vi "Swerve Drive Configs.vi"(0 "Ramp Rate":sgl, 1 "PID Constants":T1={"P Gain"=0.0, "I Gain"=0.0, "D Gain"=0.0, "F Gain"=0.0, "I Zone"=0.0, "Min Output"=-1.0, "Max Output"=1.0}, 2 "Input IDs":T4, 3 "Inversions?":T3, 4 "Idle Mode":T2) -> ()   [LabVIEW 2020]
doc: "A quick bundle to initialize all Swerve Steer motors. \nFUTURE NOTE: Consider adding individual PID controls based on performance."
uses:
  <vilib>/Rock Robotics/WPI/ThirdParty/REV Robotics/REVLib/Typedef/Spark MAX Idle Mode.ctl
  <vilib>/Rock Robotics/WPI/ThirdParty/REV Robotics/REVLib/Typedef/Spark MAX Motor Type.ctl
  <vilib>/Rock Robotics/WPI/ThirdParty/REV Robotics/REVLib/Typedef/Spark MAX Sensor Type.ctl
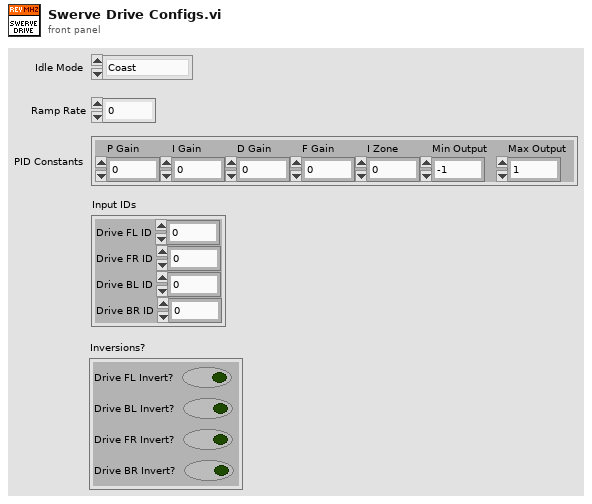
[diagram p1: front panel]
types:
  T1 = cluster{"P Gain":dbl, "I Gain":dbl, "D Gain":dbl, "F Gain":dbl, "I Zone":dbl, "Min Output":dbl, "Max Output":dbl}
  T2 = typedef "Spark MAX Idle Mode.ctl" = enum16{"Coast", "Brake"}
  T3 = cluster{"Drive FL Invert?":bool, "Drive BL Invert?":bool, "Drive FR Invert?":bool, "Drive BR Invert?":bool}
  T4 = cluster{"Drive FL ID":u8, "Drive FR ID":u8, "Drive BL ID":u8, "Drive BR ID":u8}
  T5 = typedef "Spark MAX Sensor Type.ctl" = enum16{"No Sensor", "Hall Sensor", "Encoder", "-Not Available-", "Analog", "Alternate Encoder", "Duty Cycle"}
  T6 = typedef "Spark MAX Motor Type.ctl" = enum16{"Brushed", "Brushless"}
  T7 = typedef "WPI_MotorControlDeviceRef.ctl" = cluster{"DeviceStatus":errorcluster, "Type":T8, "PWM":cluster{"PWM Channel":T9, "DeadBand":T10}, "CAN":cluster{"Device Number":u8, "SetOutput VI Ref":variant, "GetOutput VI Ref":variant, "Enable VI Ref":variant, "Disable VI Ref":variant, "Data":variant}, "Invert":bool, "DIO PWM":cluster{"PWM \"Enable\" Channel":T9, "DIOChannel":T11, "PWM Rate":dbl}}
  T8 = typedef "WPI_MotorControlType.ctl" = enum16{"PWM", "CAN", "DIO PWM"}
  T9 = typedef "FPGA_DIOPWMChannel.ctl" = enum8{"PWM 0", "PWM 1", "PWM 2", "PWM 3", "PWM 4", "PWM 5", "PWM 6", "PWM 7", "PWM 8", "PWM 9", "PWM MXP 0", "PWM MXP 1", "PWM MXP 2", "PWM MXP 3", "PWM MXP 4", "PWM MXP 5", "PWM MXP 6", "PWM MXP 7", "PWM MXP 8", "PWM MXP 9", "Invalid"}
  T10 = typedef "WPI_PWMDeadband.ctl" = cluster{"Name":string, "maxPositivePwm":i32, "minPositivePwm":i32, "centerPwm":i32, "maxNegativePwm":i32, "minNegativePwm":i32, "angularRange":u16}
  T11 = typedef "FPGA_DIOChannel.ctl" = enum8{"DIO 0", "DIO 1", "DIO 2", "DIO 3", "DIO 4", "DIO 5", "DIO 6", "DIO 7", "DIO 8", "DIO 9", "DIO MXP 0", "DIO MXP 1", "DIO MXP 2", "DIO MXP 3", "DIO MXP 4", "DIO MXP 5", "DIO MXP 6", "DIO MXP 7", "DIO MXP 8", "DIO MXP 9", "DIO MXP 10", "DIO MXP 11", "DIO MXP 12", "DIO MXP 13", "DIO MXP 14", "DIO MXP 15", "SPI Port CS1", "SPI Port CS2", "SPI Port CS3", "SPI Port MISO", "SPI Port MOSI", "Invalid"}
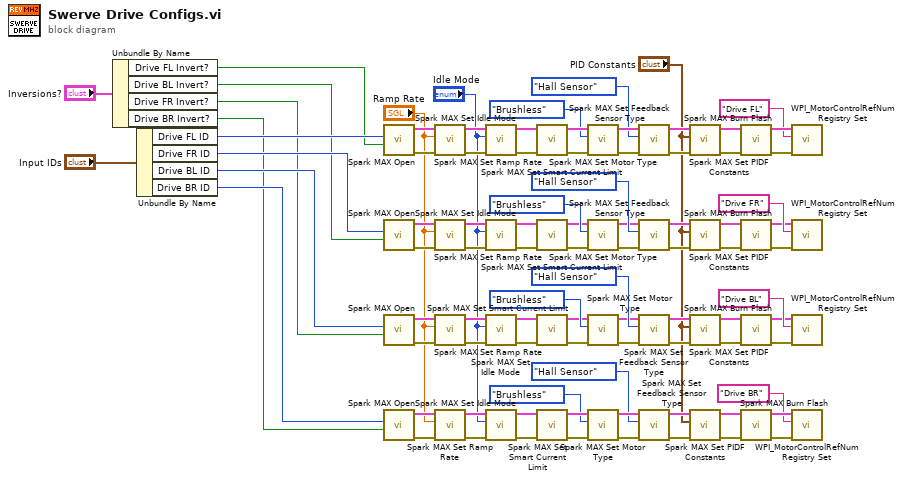
[diagram p0: block diagram]
diagram:
  n1 = Unbundle By Name("Inversions?") -> ("Drive FL Invert?"=w78:bool, "Drive BL Invert?"=w6:bool, "Drive FR Invert?"=w5:bool, "Drive BR Invert?"=w4:bool)
  n2 = Unbundle By Name("Input IDs") -> ("Drive FL ID"=w80:u8, "Drive FR ID"=w9:u8, "Drive BL ID"=w8:u8, "Drive BR ID"=w7:u8)
  n3 = call <vilib>:"Spark MAX Open.vi"("Invert"=w78, "Device Number"=w80) -> ("error out"=w67:errorcluster, "MotorControlDeviceRef"=w68:T7)  [unwired: 8 in]
  n4 = call <vilib>:"Spark MAX Open.vi"("Invert"=w6, "Device Number"=w9) -> ("error out"=w66:errorcluster, "MotorControlDeviceRef"=w65:T7)  [unwired: 8 in]
  n5 = call <vilib>:"Spark MAX Open.vi"("Invert"=w5, "Device Number"=w8) -> ("error out"=w28:errorcluster, "MotorControlDeviceRef"=w27:T7)  [unwired: 8 in]
  n6 = call <vilib>:"Spark MAX Open.vi"("Invert"=w4, "Device Number"=w7) -> ("error out"=w29:errorcluster, "MotorControlDeviceRef"=w30:T7)  [unwired: 8 in]
  n7 = call <vilib>:"Spark MAX Set Ramp Rate.vi"("error in (no error)"=w67, "Seconds from neutral to full (0)"="Ramp Rate", "MotorControlDeviceRef in"=w68) -> ("error out"=w70:errorcluster, "MotorControlDeviceRef"=w69:T7)  [unwired: 7 in]
  n8 = call <vilib>:"Spark MAX Set Ramp Rate.vi"("error in (no error)"=w66, "Seconds from neutral to full (0)"="Ramp Rate", "MotorControlDeviceRef in"=w65) -> ("error out"=w63:errorcluster, "MotorControlDeviceRef"=w64:T7)  [unwired: 7 in]
  n9 = call <vilib>:"Spark MAX Set Ramp Rate.vi"("error in (no error)"=w28, "Seconds from neutral to full (0)"="Ramp Rate", "MotorControlDeviceRef in"=w27) -> ("error out"=w25:errorcluster, "MotorControlDeviceRef"=w26:T7)  [unwired: 7 in]
  n10 = call <vilib>:"Spark MAX Set Ramp Rate.vi"("error in (no error)"=w29, "Seconds from neutral to full (0)"="Ramp Rate", "MotorControlDeviceRef in"=w30) -> ("error out"=w32:errorcluster, "MotorControlDeviceRef"=w31:T7)  [unwired: 7 in]
  n11 = call <vilib>:"Spark MAX Set Idle Mode.vi"("error in (no error)"=w70, "Idle Mode"="Idle Mode", "MotorControlDeviceRef in"=w69) -> ("error out"=w82:errorcluster, "MotorControlDeviceRef out"=w83:T7)  [unwired: 7 in]
  n12 = call <vilib>:"Spark MAX Set Idle Mode.vi"("error in (no error)"=w63, "Idle Mode"="Idle Mode", "MotorControlDeviceRef in"=w64) -> ("error out"=w55:errorcluster, "MotorControlDeviceRef out"=w54:T7)  [unwired: 7 in]
  n13 = call <vilib>:"Spark MAX Set Idle Mode.vi"("error in (no error)"=w25, "Idle Mode"="Idle Mode", "MotorControlDeviceRef in"=w26) -> ("error out"=w17:errorcluster, "MotorControlDeviceRef out"=w16:T7)  [unwired: 7 in]
  n14 = call <vilib>:"Spark MAX Set Idle Mode.vi"("error in (no error)"=w32, "Idle Mode"="Idle Mode", "MotorControlDeviceRef in"=w31) -> ("error out"=w40:errorcluster, "MotorControlDeviceRef out"=w41:T7)  [unwired: 7 in]
  n15 = call <vilib>:"Spark MAX Set Smart Current Limit.vi"("error in (no error)"=w82, "MotorControlDeviceRef in"=w83) -> ("error out"=w86:errorcluster, "MotorControlDeviceRef out"=w85:T7)  [unwired: 8 in]
  n16 = call <vilib>:"Spark MAX Set Smart Current Limit.vi"("error in (no error)"=w55, "MotorControlDeviceRef in"=w54) -> ("error out"=w51:errorcluster, "MotorControlDeviceRef out"=w52:T7)  [unwired: 8 in]
  n17 = call <vilib>:"Spark MAX Set Smart Current Limit.vi"("error in (no error)"=w17, "MotorControlDeviceRef in"=w16) -> ("error out"=w13:errorcluster, "MotorControlDeviceRef out"=w14:T7)  [unwired: 8 in]
  n18 = call <vilib>:"Spark MAX Set Smart Current Limit.vi"("error in (no error)"=w40, "MotorControlDeviceRef in"=w41) -> ("error out"=w44:errorcluster, "MotorControlDeviceRef out"=w43:T7)  [unwired: 8 in]
  n19 = call <vilib>:"Spark MAX Set Motor Type.vi"("error in (no error)"=w86, "Motor Type"=Spark_MAX_Motor_Type."Brushless", "MotorControlDevRef"=w85) -> ("error out"=w77:errorcluster, "MotorControlDeviceRef"=w76:T7)  [unwired: 7 in]
  n20 = call <vilib>:"Spark MAX Set Motor Type.vi"("error in (no error)"=w51, "Motor Type"=Spark_MAX_Motor_Type."Brushless", "MotorControlDevRef"=w52) -> ("error out"=w56:errorcluster, "MotorControlDeviceRef"=w57:T7)  [unwired: 7 in]
  n21 = call <vilib>:"Spark MAX Set Motor Type.vi"("error in (no error)"=w13, "Motor Type"=Spark_MAX_Motor_Type."Brushless", "MotorControlDevRef"=w14) -> ("error out"=w18:errorcluster, "MotorControlDeviceRef"=w19:T7)  [unwired: 7 in]
  n22 = call <vilib>:"Spark MAX Set Motor Type.vi"("error in (no error)"=w44, "Motor Type"=Spark_MAX_Motor_Type."Brushless", "MotorControlDevRef"=w43) -> ("error out"=w39:errorcluster, "MotorControlDeviceRef"=w38:T7)  [unwired: 7 in]
  n23 = call <vilib>:"Spark MAX Set Feedback Sensor Type.vi"("error in (no error)"=w77, "Sensor Type"=Spark_MAX_Sensor_Type."Hall Sensor", "MotorControlDevRef"=w76) -> ("error out"=w74:errorcluster, "MotorControlDeviceRef"=w73:T7)  [unwired: 7 in]
  n24 = call <vilib>:"Spark MAX Set Feedback Sensor Type.vi"("error in (no error)"=w56, "Sensor Type"=Spark_MAX_Sensor_Type."Hall Sensor", "MotorControlDevRef"=w57) -> ("error out"=w59:errorcluster, "MotorControlDeviceRef"=w60:T7)  [unwired: 7 in]
  n25 = call <vilib>:"Spark MAX Set Feedback Sensor Type.vi"("error in (no error)"=w18, "Sensor Type"=Spark_MAX_Sensor_Type."Hall Sensor", "MotorControlDevRef"=w19) -> ("error out"=w21:errorcluster, "MotorControlDeviceRef"=w22:T7)  [unwired: 7 in]
  n26 = call <vilib>:"Spark MAX Set Feedback Sensor Type.vi"("error in (no error)"=w39, "Sensor Type"=Spark_MAX_Sensor_Type."Hall Sensor", "MotorControlDevRef"=w38) -> ("error out"=w36:errorcluster, "MotorControlDeviceRef"=w35:T7)  [unwired: 7 in]
  n27 = call <vilib>:"Spark MAX Set PIDF Constants.vi"("error in"=w74, "PID Constants"="PID Constants", "MotorControlDeviceRef"=w73) -> ("error out"=w71:errorcluster, "MotorControlDeviceRef"=w72:T7)  [unwired: 7 in]
  n28 = call <vilib>:"Spark MAX Set PIDF Constants.vi"("error in"=w59, "PID Constants"="PID Constants", "MotorControlDeviceRef"=w60) -> ("error out"=w62:errorcluster, "MotorControlDeviceRef"=w61:T7)  [unwired: 7 in]
  n29 = call <vilib>:"Spark MAX Set PIDF Constants.vi"("error in"=w21, "PID Constants"="PID Constants", "MotorControlDeviceRef"=w22) -> ("error out"=w24:errorcluster, "MotorControlDeviceRef"=w23:T7)  [unwired: 7 in]
  n30 = call <vilib>:"Spark MAX Set PIDF Constants.vi"("error in"=w36, "PID Constants"="PID Constants", "MotorControlDeviceRef"=w35) -> ("error out"=w33:errorcluster, "MotorControlDeviceRef"=w34:T7)  [unwired: 7 in]
  n31 = call <vilib>:"Spark MAX Burn Flash.vi"("error in"=w71, "MotorControlDeviceRef"=w72) -> ("error out"=w89:errorcluster, "MotorControlDeviceRef"=w88:T7)  [unwired: 8 in]
  n32 = call <vilib>:"Spark MAX Burn Flash.vi"("error in"=w62, "MotorControlDeviceRef"=w61) -> ("error out"=w48:errorcluster, "MotorControlDeviceRef"=w49:T7)  [unwired: 8 in]
  n33 = call <vilib>:"Spark MAX Burn Flash.vi"("error in"=w24, "MotorControlDeviceRef"=w23) -> ("error out"=w10:errorcluster, "MotorControlDeviceRef"=w11:T7)  [unwired: 8 in]
  n34 = call <vilib>:"Spark MAX Burn Flash.vi"("error in"=w33, "MotorControlDeviceRef"=w34) -> ("error out"=w47:errorcluster, "MotorControlDeviceRef"=w46:T7)  [unwired: 8 in]
  n35 = call <vilib>:"WPI_MotorControlRefNum Registry Set.vi"("error in (no error)"=w89, "refnum name"="Drive FL" ("Change to match from begin.vi"), "MotorControlDevRef"=w88) -> ()  [unwired: 7 in, 2 out]
  n36 = call <vilib>:"WPI_MotorControlRefNum Registry Set.vi"("error in (no error)"=w48, "refnum name"="Drive FR" ("Change to match from begin.vi"), "MotorControlDevRef"=w49) -> ()  [unwired: 7 in, 2 out]
  n37 = call <vilib>:"WPI_MotorControlRefNum Registry Set.vi"("error in (no error)"=w10, "refnum name"="Drive BL" ("Change to match from begin.vi"), "MotorControlDevRef"=w11) -> ()  [unwired: 7 in, 2 out]
  n38 = call <vilib>:"WPI_MotorControlRefNum Registry Set.vi"("error in (no error)"=w47, "refnum name"="Drive BR" ("Change to match from begin.vi"), "MotorControlDevRef"=w46) -> ()  [unwired: 7 in, 2 out]
